vi "TPD Demonstrator.vi"() -> ()   [LabVIEW 2011]
uses:
  <vilib>/ptbypt/NI_PtbyPt.lvlib
panel:
  in  "Tol":dbl=0.12 step=0.01
  out "Up ?":bool
  out "Waveform Chart":cluster{dbl, dbl, dbl, dbl, dbl}(graph)
  in  "reset":bool
  out "I+N":dbl
  in  "Input":dbl step=0.1
  in  "Manual":bool
  in  "amplitude":dbl=0.9999999999999999 step=0.1 format="%0.2f"
  in  "frequency":dbl=0.0001 format="%0.4e"
  in  "Use Time ?":bool=TRUE
  in  "noise":dbl(knob)=0.05940857995844632 scale=0.0..0.1
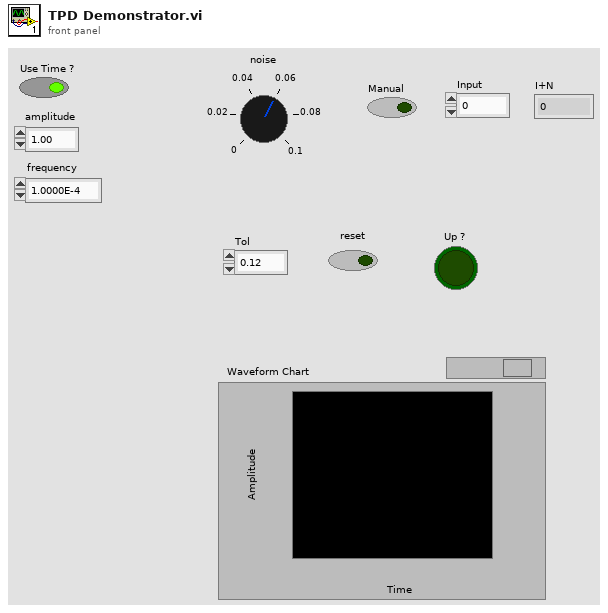
[diagram p1: front panel]
types:
  T1 = cluster{dbl, "Local Hi Peak":dbl, "Local Lo Peak":dbl, "Global Hi Peak":dbl, "Global Lo Peak":dbl}
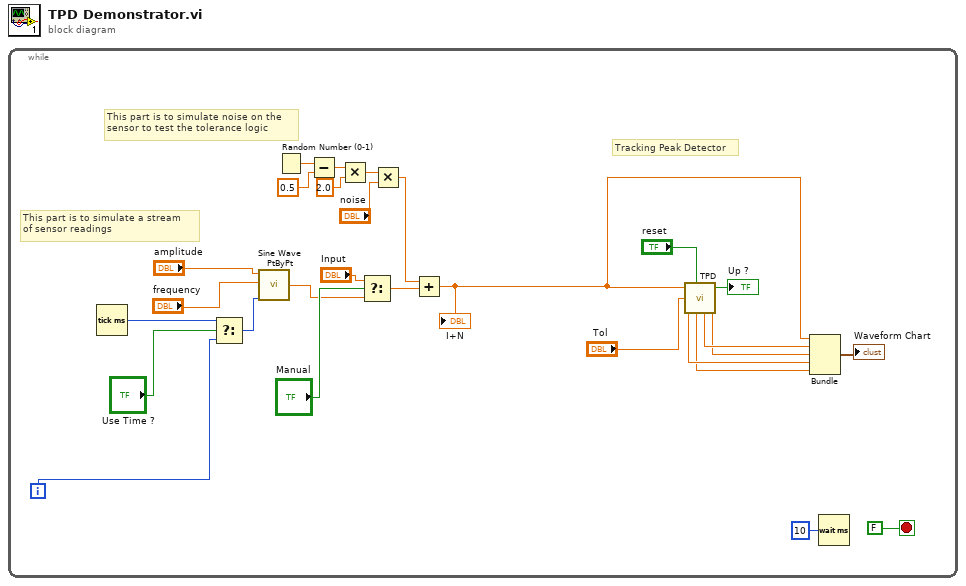
[diagram p0: block diagram]
diagram:
  n1 = while {
    i -> [w23]
    stop <- FALSE stop-if-true
    # "Tracking Peak Detector"
    # "This part is to simulate noise on the \nsensor to test the tolerance logic"
    # "This part is to simulate a stream\nof sensor readings"
    n2 = Tick Count (ms)() -> (millisecond timer value=w26:u32)
    n3 = Select(t=w26, s="Use Time ?", f=w23) -> (s? t:f=w25:u32)
    n4 = call <vilib>:"Sine Wave PtByPt.vi"("time"=w25, "frequency"="frequency", "amplitude"="amplitude") -> ("sine wave"=w11:dbl)  [unwired: 1 in]
    n5 = Random Number (0-1)() -> (number: 0 to 1=w20:dbl)
    n6 = Subtract(x=w20, y=0.5) -> (x-y=w18:dbl)
    n7 = Multiply(x=w18, y=2.0) -> (x*y=w16:dbl)
    n8 = Select(t="Input", s="Manual", f=w11) -> (s? t:f=w13:dbl)
    n9 = Multiply(x=w16, y="noise") -> (x*y=w14:dbl)
    n10 = Add(x=w14, y=w13) -> (x+y=w7:dbl)
    "I+N" <- w7
    n11 = call "TPD.vi"("Input"=w7, "reset"="reset", "Tol"="Tol") -> ("Global Hi Peak"=w4:dbl, "Global Lo Peak"=w3:dbl, "Up ?"=→"Up ?":bool, "Local Hi Peak"=w6:dbl, "Local Lo Peak"=w5:dbl)  [unwired: 2 in]
    n12 = Bundle(w7, "Local Hi Peak"=w6, "Local Lo Peak"=w5, "Global Hi Peak"=w4, "Global Lo Peak"=w3) -> (→"Waveform Chart":T1)  [unwired: 1 in]
    n13 = Wait (ms)(milliseconds to wait=u32 10) -> ()  [unwired: 1 out]
  }
